vi "Profile Auton - Angle.vi"(8 "error in (no error)":errorcluster, 10 "Time (s)":dbl, 11 "Angle (degrees)":dbl) -> (0 "error out":errorcluster)   [LabVIEW 2017]
uses:
  Robot Global Data.vi
  <vilib>/Rock Robotics/Network Tables/NT Write Number.vi
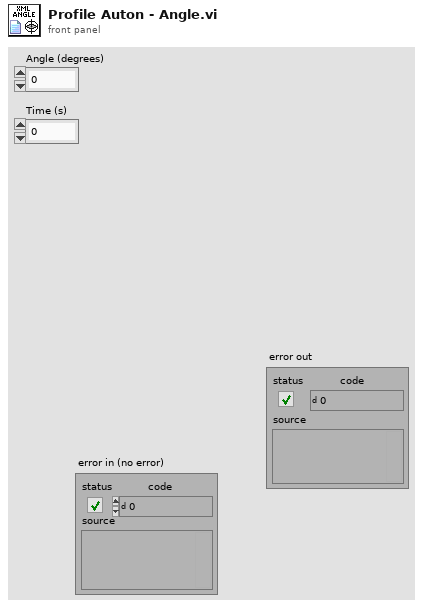
[diagram p1: front panel]
types:
  T1 = typedef "WPI_RobotDriveDevRef.ctl" = cluster{"DevStatus":errorcluster, "Motors[]":T2[], "Square Inputs":bool, "Max Output":dbl}
  T2 = typedef "WPI_MotorControlDeviceRef.ctl" = cluster{"DeviceStatus":errorcluster, "Type":T3, "PWM":cluster{"PWM Channel":T4, "DeadBand":T5}, "CAN":cluster{"Device Number":u8, "SetOutput VI Ref":variant, "GetOutput VI Ref":variant, "Enable VI Ref":variant, "Disable VI Ref":variant, "Data":variant}, "Invert":bool, "DIO PWM":cluster{"PWM \"Enable\" Channel":T4, "DIOChannel":T6, "PWM Rate":dbl}}
  T3 = typedef "WPI_MotorControlType.ctl" = enum16{"PWM", "CAN", "DIO PWM"}
  T4 = typedef "FPGA_DIOPWMChannel.ctl" = enum8{"PWM 0", "PWM 1", "PWM 2", "PWM 3", "PWM 4", "PWM 5", "PWM 6", "PWM 7", "PWM 8", "PWM 9", "PWM MXP 0", "PWM MXP 1", "PWM MXP 2", "PWM MXP 3", "PWM MXP 4", "PWM MXP 5", "PWM MXP 6", "PWM MXP 7", "PWM MXP 8", "PWM MXP 9", "Invalid"}
  T5 = typedef "WPI_PWMDeadband.ctl" = cluster{"Name":string, "maxPositivePwm":i32, "minPositivePwm":i32, "centerPwm":i32, "maxNegativePwm":i32, "minNegativePwm":i32, "angularRange":u16}
  T6 = typedef "FPGA_DIOChannel.ctl" = enum8{"DIO 0", "DIO 1", "DIO 2", "DIO 3", "DIO 4", "DIO 5", "DIO 6", "DIO 7", "DIO 8", "DIO 9", "DIO MXP 0", "DIO MXP 1", "DIO MXP 2", "DIO MXP 3", "DIO MXP 4", "DIO MXP 5", "DIO MXP 6", "DIO MXP 7", "DIO MXP 8", "DIO MXP 9", "DIO MXP 10", "DIO MXP 11", "DIO MXP 12", "DIO MXP 13", "DIO MXP 14", "DIO MXP 15", "SPI Port CS1", "SPI Port CS2", "SPI Port CS3", "SPI Port MISO", "SPI Port MOSI", "Invalid"}
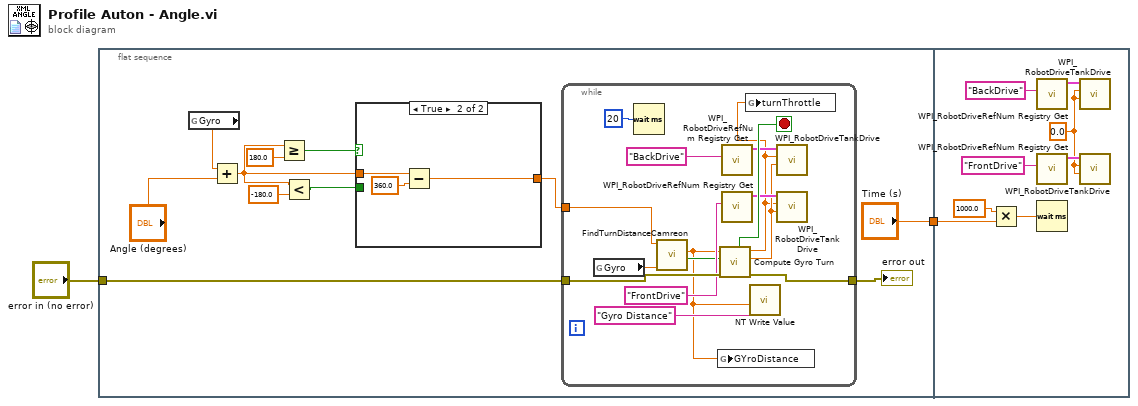
[diagram p0: block diagram]
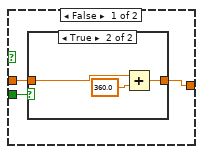
[diagram p2: hidden frame]
diagram:
  n1 = flat-sequence {
    tunnel: ["Time (s)"] -> w2
    tunnel: "error in (no error)" -> [w11]
    tunnel: w2 -> [w44]
    frame #0 {
      n2 = global read "Robot Global Data.vi" "Gyro"() -> (w10:dbl)
      n3 = Add(x=w10, y="Angle (degrees)") -> (x+y=w4:dbl)
      n4 = Greater Or Equal?(x=w4, y=180.0 ("x")) -> (x >= y?=w9:bool)
      n5 = Less?(x=w4, y=-180.0 ("x")) -> (x < y?=w5:bool)
      n6 = case shown="True" w9 {
        tunnel: w4 -> [w14 w23]
        tunnel: w5 -> [w16 _]
        tunnel: [w15 w21] -> w7
        frame False {
          n7 = case shown="True" w16 {
            tunnel: [w17 w20] -> w15
            tunnel: w14 -> [w17 w19]
            frame False {
            }
            frame True {
              n8 = Add(x=w19, y=360.0 ("x")) -> (x+y=w20:dbl)
            }
          }
        }
        frame True {
          n9 = Subtract(x=w23, y=360.0 ("x")) -> (x-y=w21:dbl)
        }
      }
      n10 = while {
        tunnel: [w36] -> w13
        tunnel: w11 -> [w35]
        tunnel: w7 -> [w29]
        stop <- w37 stop-if-true
        n11 = global read "Robot Global Data.vi" "Gyro"() -> (w28:dbl)
        n12 = Wait (ms)(milliseconds to wait=u32 20) -> ()  [unwired: 1 out]
        n13 = call "FindTurnDistanceCamreon.vi"("Current"=w28, "Wanted"=w29) -> ("Negate"=w26:bool, "Distance"=w25:dbl)  [unwired: 8 in]
        n14 = global write "Robot Global Data.vi" "GYroDistance"(w25) -> ()
        n15 = call "Compute Gyro Turn.vi"("error in (no error)"=w35, "Negate stuff"=w26, "Turn? Right Positive."=w25) -> ("error out"=w36:errorcluster, "Right Drive"=w30:dbl, "Left drive"=w24:dbl, "done"=w37:bool)  [unwired: 5 in]
        n16 = call <vilib>:"WPI_RobotDriveRefNum Registry Get.vi"("refnum name"="BackDrive") -> ("RobotDriveDevRef"=w33:T1)  [unwired: 9 in, 1 out]
        n17 = call <vilib>:"WPI_RobotDriveRefNum Registry Get.vi"("refnum name"="FrontDrive") -> ("RobotDriveDevRef"=w34:T1)  [unwired: 9 in, 1 out]
        n18 = global write "Robot Global Data.vi" "turnThrottle"(w24) -> ()
        n19 = call-poly <vilib>:"NT Write Value.vi"("Numeric"=w25, "Name"="Gyro Distance") -> ()  [unwired: 9 in, 1 out]
        n20 = call <vilib>:"WPI_RobotDriveTankDrive.vi"("Right axis value"=w30, "Left axis value"=w24, "RobotDriveDevRef"=w33) -> ()  [unwired: 6 in, 3 out]
        n21 = call <vilib>:"WPI_RobotDriveTankDrive.vi"("Right axis value"=w30, "Left axis value"=w24, "RobotDriveDevRef"=w34) -> ()  [unwired: 6 in, 3 out]
      }
      "error out" <- w13
    }
    frame #1 {
      w39 = 0.0
      n22 = Multiply(x=1000.0, y=w44) -> (x*y=w46:dbl)
      n23 = call <vilib>:"WPI_RobotDriveRefNum Registry Get.vi"("refnum name"="BackDrive") -> ("RobotDriveDevRef"=w41:T1)  [unwired: 9 in, 1 out]
      n24 = call <vilib>:"WPI_RobotDriveRefNum Registry Get.vi"("refnum name"="FrontDrive") -> ("RobotDriveDevRef"=w40:T1)  [unwired: 9 in, 1 out]
      n25 = Wait (ms)(milliseconds to wait=w46) -> ()  [unwired: 1 out]
      n26 = call <vilib>:"WPI_RobotDriveTankDrive.vi"("Right axis value"=w39, "Left axis value"=w39, "RobotDriveDevRef"=w41) -> ()  [unwired: 6 in, 3 out]
      n27 = call <vilib>:"WPI_RobotDriveTankDrive.vi"("Right axis value"=w39, "Left axis value"=w39, "RobotDriveDevRef"=w40) -> ()  [unwired: 6 in, 3 out]
    }
  }
